vi "GetObstacleData.vi"(8 "error in (no error)":errorcluster, 11 "Obstacle.lvclass":refnum<class "Obstacle.lvclass">) -> (0 "error out":errorcluster, 1 "List of Line Segments in Obstacle":T2(array[cluster]) {"UTM Obstacle Point 2"."North" format="%#_10f"; "UTM Obstacle Point 2"."East" format="%#_8f"; "UTM Obstacle Point 1"."North" format="%#_10f"; "UTM Obstacle Point 1"."East" format="%#_8f"}, 2 "ID#":i32, 3 "Obstacle":refnum<class "Obstacle.lvclass">)   [LabVIEW 2013, in "Obstacle.lvclass"]
doc: "This VI outputs the internal variables of the obstacle object.\n\nEric Schneider, August 2014"
uses:
  Obstacle.lvclass
  Data/TypeDefs/UTM Location.ctl
  Obstacle.lvclass/Obstacle.ctl
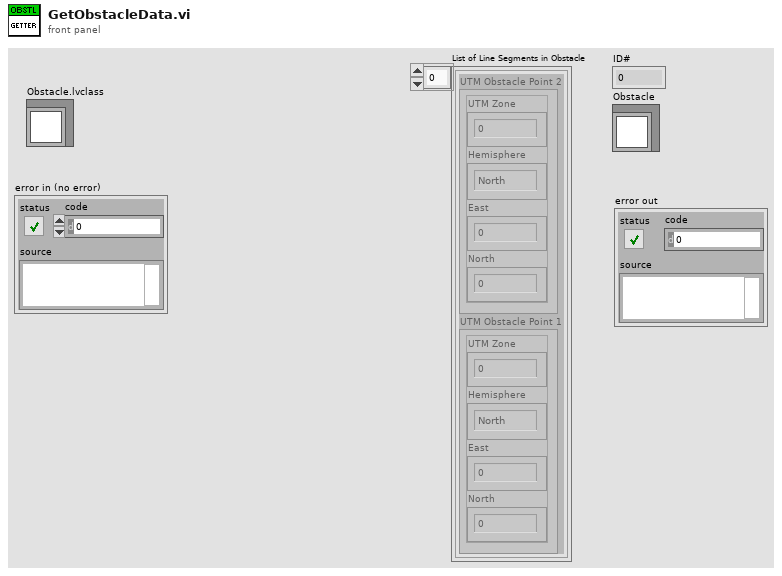
[diagram p1: front panel]
types:
  T1 = typedef "UTM Location.ctl" = cluster{"UTM Zone":dbl, "Hemisphere":enum16{"North", "South"}, "East":dbl, "North":dbl}
  T2 = cluster{"UTM Obstacle Point 2":T1, "UTM Obstacle Point 1":T1}[]
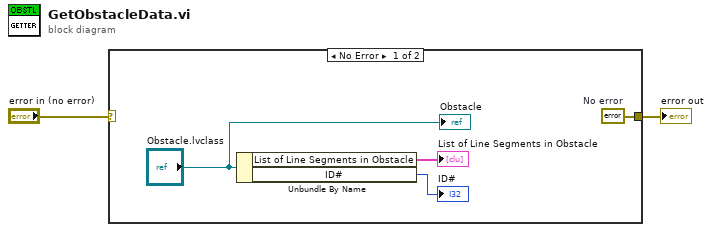
[diagram p0: block diagram]
diagram:
  n1 = case shown="No Error" "error in (no error)" {
    selector: "error in (no error)" -> [_ w7]
    tunnel: [w3 w7] -> w1
    frame No Error {
      w3 = errorcluster {"status"=FALSE, "code"=0, "source"=""}  # No error
      n2 = Unbundle By Name("Obstacle.lvclass") -> ("List of Line Segments in Obstacle"=→"List of Line Segments in Obstacle":T2, "ID#"=→"ID#":i32)
      "Obstacle" <- "Obstacle.lvclass"
    }
    frame Error {
    }
  }
  "error out" <- w1
